vi "SaveReadPrefs.vi"(3 "Task":enum16{"Read", "Save"}(ring)) -> (0 "Masters":string[](array[string]))   [LabVIEW 2016]
doc: "Reads or saves preferences to the Master History global"
uses:
  _ROSDefinition.vi
panel:
  out "error out":errorcluster
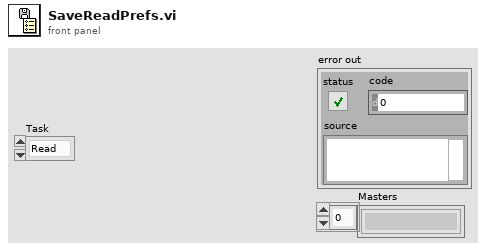
[diagram p1: front panel]
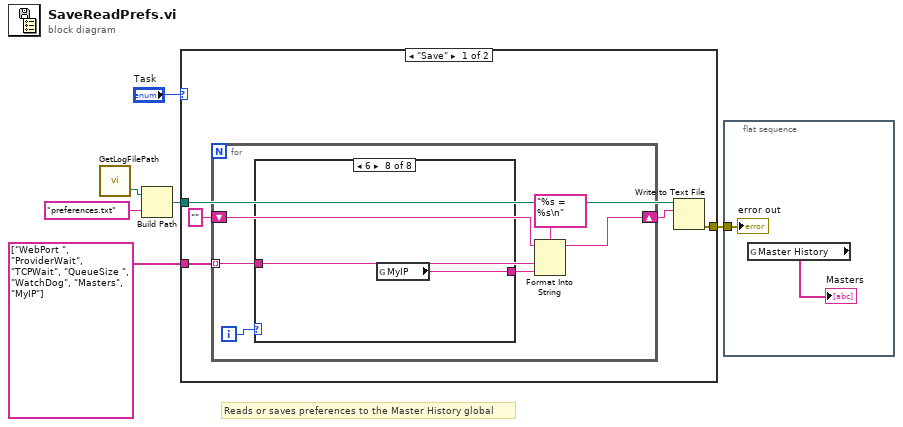
[diagram p0: block diagram]
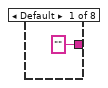
[diagram p2: hidden frame]
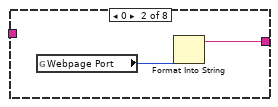
[diagram p3: hidden frame]
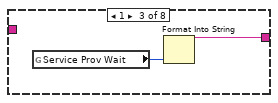
[diagram p4: hidden frame]
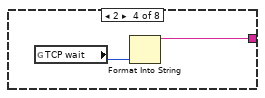
[diagram p5: hidden frame]
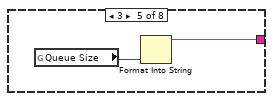
[diagram p6: hidden frame]
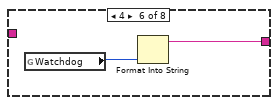
[diagram p7: hidden frame]
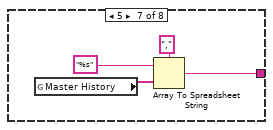
[diagram p8: hidden frame]
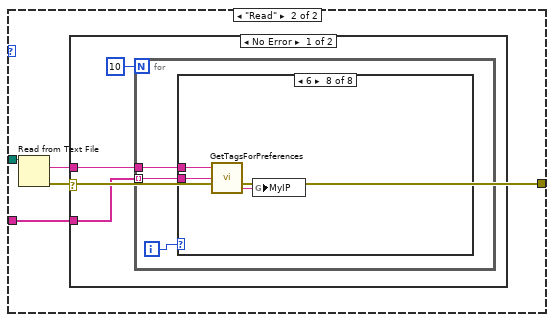
[diagram p9: hidden frame]
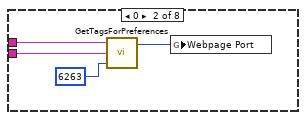
[diagram p11: hidden frame]
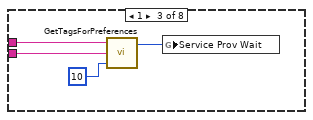
[diagram p12: hidden frame]
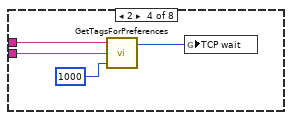
[diagram p13: hidden frame]
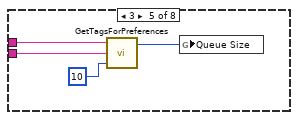
[diagram p14: hidden frame]
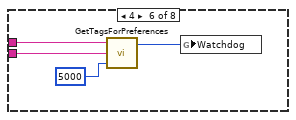
[diagram p15: hidden frame]
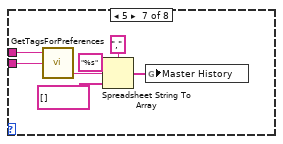
[diagram p16: hidden frame]
diagram:
  # "Reads or saves preferences to the Master History global"
  n1 = call "GetLogFilePath.vi"() -> ("LogFolder"=w6:path)  [unwired: 2 in, 1 out]
  n2 = Build Path(base path=w6, name or relative path="preferences.txt") -> (appended path=w4:path)
  n3 = case shown="\"Save\"" "Task" {
    tunnel: w4 -> [w9 w37]
    tunnel: string[] ["WebPort ", "ProviderWait", "TCPWait", "QueueSize ", "WatchDog", "Masters", "MyIP"] -> [w11 w35]
    tunnel: [w8 w34] -> w1
    frame "Save" {
      n4 = for {
        tunnel: w11 -> [w15] mode=indexing
        shift-right: [w13] -> w10
        shift-left: "" -> [w12]
        i -> [w17]
        n5 = case shown="6" w17 {
          tunnel: w15 -> [_ _ _ _ _ _ _ _]
          tunnel: ["" ("spreadsheet string") w19 w22 w24 w26 w28 w29 w33] -> w14
          frame Default {
          }
          frame 0 {
            n6 = global read "_ROSDefinition.vi" "Webpage Port"() -> (w20:u16)
            n7 = Format Into String(w20) -> (resulting string=w19:string)  [unwired: 3 in, 1 out]
          }
          frame 1 {
            n8 = global read "_ROSDefinition.vi" "Service Prov Wait"() -> (w21:i32)
            n9 = Format Into String(w21) -> (resulting string=w22:string)  [unwired: 3 in, 1 out]
          }
          frame 2 {
            n10 = global read "_ROSDefinition.vi" "TCP wait"() -> (w23:i32)
            n11 = Format Into String(w23) -> (resulting string=w24:string)  [unwired: 3 in, 1 out]
          }
          frame 3 {
            n12 = global read "_ROSDefinition.vi" "Queue Size"() -> (w25:i32)
            n13 = Format Into String(w25) -> (resulting string=w26:string)  [unwired: 3 in, 1 out]
          }
          frame 4 {
            n14 = global read "_ROSDefinition.vi" "Watchdog"() -> (w27:i32)
            n15 = Format Into String(w27) -> (resulting string=w28:string)  [unwired: 3 in, 1 out]
          }
          frame 5 {
            n16 = global read "_ROSDefinition.vi" "Master History"() -> (w32:string[])
            n17 = Array To Spreadsheet String(delimiter (Tab)=",", array=w32, 3:"%s" ("format string")) -> (spreadsheet string=w29:string)
          }
          frame 6 {
            n18 = global read "_ROSDefinition.vi" "MyIP"() -> (w33:string)
          }
        }
        n19 = Format Into String(format string="%s = %s\n", initial string=w12, w15, w14) -> (resulting string=w13:string)  [unwired: 1 in, 1 out]
      }
      n20 = Write to Text File(file (use dialog)=w9, text=w10) -> (error out=w8:errorcluster)  [unwired: 2 in, 2 out]
    }
    frame "Read" {
      n21 = Read from Text File(file (use dialog)=w37) -> (text=w36:string, error out=w34:errorcluster)  [unwired: 3 in, 2 out]
      n22 = case shown="No Error" w34 {
        tunnel: w36 -> [w39 _]
        tunnel: w35 -> [w38 _]
        frame No Error {
          n23 = for {
            N: 10 -> [_]
            tunnel: w39 -> [w42]
            tunnel: w38 -> [w41] mode=indexing
            i -> [w43]
            n24 = case shown="6" w43 {
              tunnel: w42 -> [_ w47 w51 w55 w59 w63 w70 w73]
              tunnel: w41 -> [_ w44 w48 w52 w56 w60 w69 w72]
              frame Default {
              }
              frame 0 {
                n25 = call "GetTagsForPreferences.vi"("Default"=u16 6263 ("t"), "Tag"=w44, "File"=w47) -> ("tag value"=w45:i32)  [unwired: 1 in, 1 out]
                n26 = global write "_ROSDefinition.vi" "Webpage Port"(w45) -> ()
              }
              frame 1 {
                n27 = call "GetTagsForPreferences.vi"("Default"=u16 10 ("t"), "Tag"=w48, "File"=w51) -> ("tag value"=w49:i32)  [unwired: 1 in, 1 out]
                n28 = global write "_ROSDefinition.vi" "Service Prov Wait"(w49) -> ()
              }
              frame 2 {
                n29 = call "GetTagsForPreferences.vi"("Default"=u16 1000 ("t"), "Tag"=w52, "File"=w55) -> ("tag value"=w53:i32)  [unwired: 1 in, 1 out]
                n30 = global write "_ROSDefinition.vi" "TCP wait"(w53) -> ()
              }
              frame 3 {
                n31 = call "GetTagsForPreferences.vi"("Default"=u16 10 ("t"), "Tag"=w56, "File"=w59) -> ("tag value"=w57:i32)  [unwired: 1 in, 1 out]
                n32 = global write "_ROSDefinition.vi" "Queue Size"(w57) -> ()
              }
              frame 4 {
                n33 = call "GetTagsForPreferences.vi"("Default"=u16 5000 ("t"), "Tag"=w60, "File"=w63) -> ("tag value"=w61:i32)  [unwired: 1 in, 1 out]
                n34 = global write "_ROSDefinition.vi" "Watchdog"(w61) -> ()
              }
              frame 5 {
                n35 = call "GetTagsForPreferences.vi"("Tag"=w69, "File"=w70) -> ("tag"=w67:string)  [unwired: 2 in, 1 out]
                n36 = Spreadsheet String To Array(delimiter (Tab)=",", format string="%s", spreadsheet string=w67, array type (2D Dbl)=string[] [] ("Master History")) -> (array=w65:string[])
                n37 = global write "_ROSDefinition.vi" "Master History"(w65) -> ()
              }
              frame 6 {
                n38 = call "GetTagsForPreferences.vi"("Tag"=w72, "File"=w73) -> ("tag"=w71:string)  [unwired: 2 in, 1 out]
                n39 = global write "_ROSDefinition.vi" "MyIP"(w71) -> ()
              }
            }
          }
        }
        frame Error {
        }
      }
    }
  }
  n40 = flat-sequence {
    tunnel: w1 -> [w75]
    frame #0 {
      n41 = global read "_ROSDefinition.vi" "Master History"() -> (→"Masters":string[])
      "error out" <- w75
    }
  }
